vi "Demodulacja_DSBSC.vi"(0 "Sygnal_zmodulowany":dbl[](array[numeric]), 1 "Pasmo_przenoszenia":cluster{"f_L":dbl, "f_H":dbl}, 2 "Czestotliwosc_probkowania":dbl, 3 "Czas":dbl, 4 "Parametry_sygnalu_nosnego":T1) -> (7 "Sygnal_zdemodulowany":dbl[](array[numeric]))   [LabVIEW 2020]
doc: "VI demoduluje sygnal zmodulowany metoda DSBSC"
uses:
  Kontrolki/Parametry_cosinusa.ctl
  <vilib>/Analysis/3filter.llb/Filter Passband Type.ctl
  <vilib>/Analysis/3filter.llb/Butterworth Filter (DBL).vi
  <vilib>/Analysis/NI_AALBase.lvlib
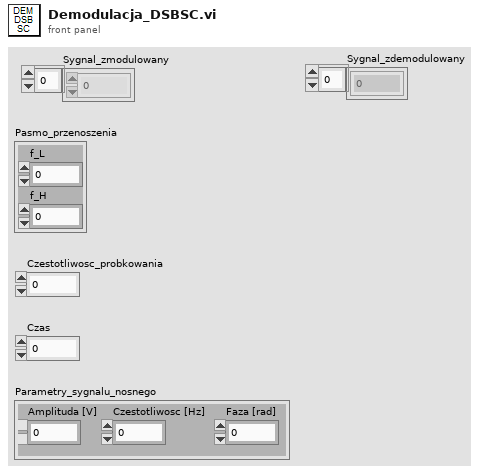
[diagram p1: front panel]
types:
  T1 = typedef "Parametry_cosinusa.ctl" = cluster{"Amplituda [V]":dbl, "Czestotliwosc [Hz] ":dbl, "Faza [rad]":dbl}
  T2 = typedef "NI_AALBase.lvlib/Filter Passband Type.ctl" = enum32{"Lowpass", "Highpass", "Bandpass", "Bandstop"}
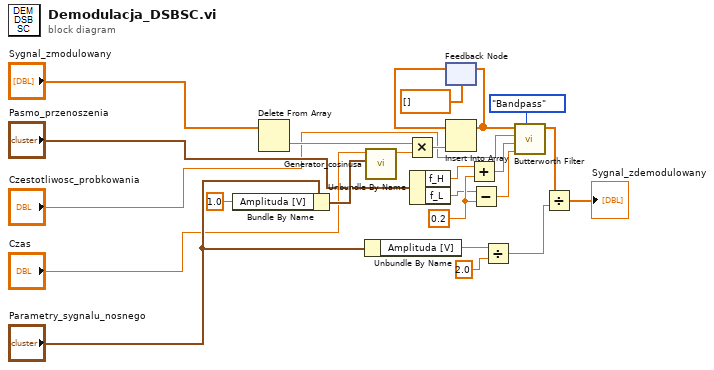
[diagram p0: block diagram]
diagram:
  w14 = 0.2
  n1 = Bundle By Name(cluster="Parametry_sygnalu_nosnego", "Amplituda [V]"=1.0) -> (w18:T1)
  n2 = Delete From Array(array="Sygnal_zmodulowany") -> (deleted portion=w7:dbl)  [unwired: 2 in, 1 out]
  n3 = Unbundle By Name("Parametry_sygnalu_nosnego") -> ("Amplituda [V]"=w19:dbl)
  n4 = call "Generator_cosinusa.vi"("Parametry_cosinusa"=w18, "Czas"="Czas") -> ("A cos(2pift + phi)"=w5:dbl)  [unwired: 9 in]
  n5 = Multiply(x=w7, y=w5) -> (x*y=w8:dbl)
  n6 = Unbundle By Name("Pasmo_przenoszenia") -> ("f_H"=w12:dbl, "f_L"=w13:dbl)
  n7 = feedback #1(dbl[] []) -> (w10:dbl[])
  n8 = Insert Into Array(array=w10, new element=w8) -> (w11:dbl[])  [unwired: 1 in]
  n9 = feedback-in #1(w11) -> ()
  n10 = Add(x=w12, y=w14) -> (x+y=w15:dbl)
  n11 = Subtract(x=w13, y=w14) -> (x-y=w16:dbl)
  n12 = Divide(x=w19, y=2.0) -> (x/y=w21:dbl)
  n13 = call-poly <vilib>:"Butterworth Filter.vi"("filter type"=Filter_Passband_Type."Bandpass", "low cutoff freq: fl"=w16, "high cutoff freq: fh"=w15, "sampling freq: fs"="Czestotliwosc_probkowania", "X"=w11) -> ("Filtered X"=w22:dbl[])  [unwired: 3 in, 1 out]
  n14 = Divide(x=w22, y=w21) -> (x/y=→"Sygnal_zdemodulowany":dbl[])
